vi "Timeout Manager.vi"(8 "error in (no error)":errorcluster, 11 "bt_WaitOn_Synch in":refnum<class "bt_WaitOn_Synch.lvclass">) -> (0 "error out":errorcluster, 1 "Timeout":i32, 2 "Timeout Now?":bool, 3 "bt_WaitOn_Synch out":refnum<class "bt_WaitOn_Synch.lvclass">)   [LabVIEW 2021, in "BT.lvlib" / "bt_WaitOn_Synch.lvclass"]
uses:
  bt_WaitOn_Synch.lvclass
  bt_WaitOn_Synch.lvclass/bt_WaitOn_Synch.ctl
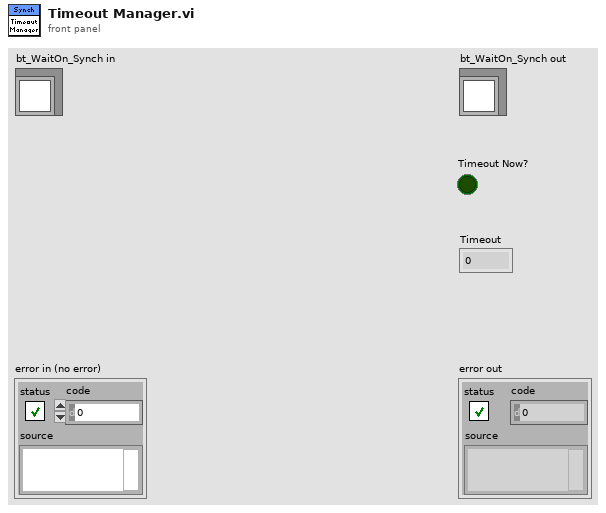
[diagram p1: front panel]
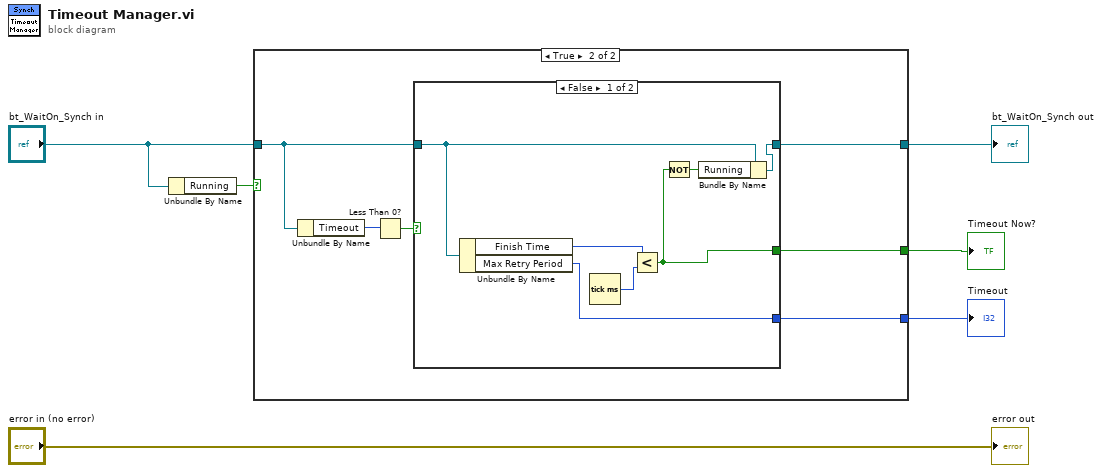
[diagram p0: block diagram]
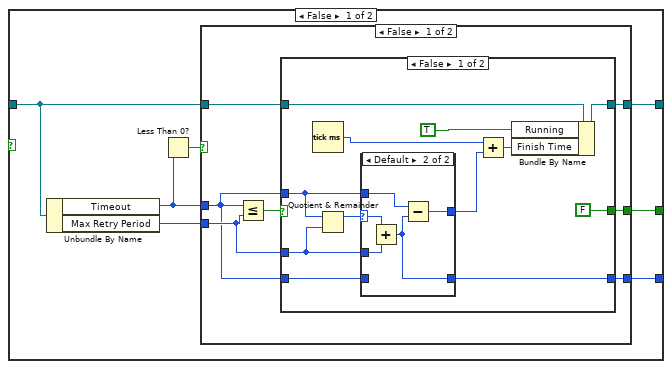
[diagram p2: hidden frame]
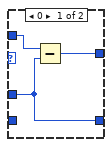
[diagram p3: hidden frame]
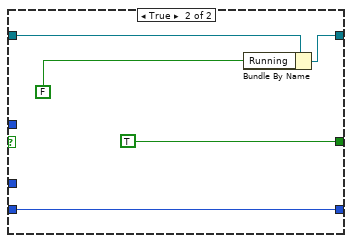
[diagram p4: hidden frame]
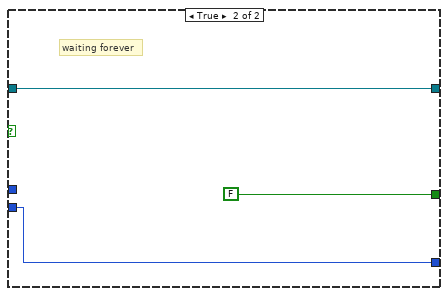
[diagram p5: hidden frame]
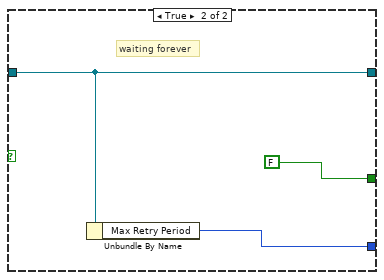
[diagram p6: hidden frame]
diagram:
  n1 = Unbundle By Name("bt_WaitOn_Synch in") -> ("Running"=w5:bool)
  n2 = case shown="True" w5 {
    tunnel: "bt_WaitOn_Synch in" -> [w12 w52]
    tunnel: [w13 w51] -> w3
    tunnel: [w11 w50] -> w2
    tunnel: [w10 w49] -> w1
    frame False {
      n3 = Unbundle By Name(w12) -> ("Timeout"=w7:i32, "Max Retry Period"=w9:i32)
      n4 = Less Than 0?(x=w7) -> (x < 0?=w8:bool)
      n5 = case shown="False" w8 {
        tunnel: [w20 w48] -> w13
        tunnel: w12 -> [w19 w48]
        tunnel: [w17 FALSE] -> w11
        tunnel: [w16 w46] -> w10
        tunnel: w7 -> [w14 _]
        tunnel: w9 -> [w15 w46]
        frame False {
          n6 = Less Or Equal?(x=w14, y=w15) -> (x <= y?=w18:bool)
          n7 = case shown="False" w18 {
            tunnel: [w31 w45] -> w20
            tunnel: w19 -> [w32 w44]
            tunnel: [FALSE TRUE] -> w17
            tunnel: [w25 w41] -> w16
            tunnel: w14 -> [w24 w41]
            tunnel: w15 -> [w23 _]
            tunnel: w14 -> [w22 _]
            frame False {
              n8 = Tick Count (ms)() -> (millisecond timer value=w28:u32)
              n9 = Quotient & Remainder(x=w22, y=w23) -> (x-y*floor(x/y)=w26:i32)  [unwired: 1 out]
              n10 = case shown="Default" w26 {
                selector: w26 -> [_ w38]
                tunnel: [w34 w36] -> w25
                tunnel: w24 -> [_ _]
                tunnel: w23 -> [w34 w37]
                tunnel: w22 -> [w35 w39]
                tunnel: [w33 w40] -> w21
                frame 0 {
                  n11 = Subtract(x=w35, y=w34) -> (x-y=w33:i32)
                }
                frame Default {
                  n12 = Add(x=w38, y=w37) -> (x+y=w36:i32)
                  n13 = Subtract(x=w39, y=w36) -> (x-y=w40:i32)
                }
              }
              n14 = Add(x=w28, y=w21) -> (x+y=w27:u32)
              n15 = Bundle By Name(cluster=w32, "Running"=TRUE, "Finish Time"=w27) -> (w31:refnum<class "bt_WaitOn_Synch.lvclass">)
            }
            frame True {
              n16 = Bundle By Name(cluster=w44, "Running"=FALSE) -> (w45:refnum<class "bt_WaitOn_Synch.lvclass">)
            }
          }
        }
        frame True {
          # "waiting forever"
        }
      }
    }
    frame True {
      n17 = Unbundle By Name(w52) -> ("Timeout"=w54:i32)
      n18 = Less Than 0?(x=w54) -> (x < 0?=w53:bool)
      n19 = case shown="False" w53 {
        tunnel: w52 -> [w58 w64]
        tunnel: [w57 w64] -> w51
        tunnel: [w55 FALSE] -> w50
        tunnel: [w59 w62] -> w49
        frame False {
          n20 = Unbundle By Name(w58) -> ("Finish Time"=w61:u32, "Max Retry Period"=w59:i32)
          n21 = Tick Count (ms)() -> (millisecond timer value=w60:u32)
          n22 = Less?(x=w61, y=w60) -> (x < y?=w55:bool)
          n23 = Not(x=w55) -> (.not. x?=w56:bool)
          n24 = Bundle By Name(cluster=w58, "Running"=w56) -> (w57:refnum<class "bt_WaitOn_Synch.lvclass">)
        }
        frame True {
          # "waiting forever"
          n25 = Unbundle By Name(w64) -> ("Max Retry Period"=w62:i32)
        }
      }
    }
  }
  "bt_WaitOn_Synch out" <- w3
  "Timeout Now?" <- w2
  "Timeout" <- w1
  "error out" <- "error in (no error)"
